vi "SV TDMS Write Octave (1 Ch).vi"(0 "tdms file":refnum<k34>, 5 "group name in":string="Octave", 7 "channel name in":string="Channel0", 9 "octave spectrum":T1, 11 "error in":errorcluster, 13 "octave info":T2={"standard"=enum."ANSI S1.11", "bandwidth"=enum."1 octave", "low band"=0, "high band"=0, "weighting filter"=0, "dB reference"=0.0, "dB On"=FALSE, "unit label"="", "channel name"="", "description"="", "engineering units"=1, "custom label"="", "spectrum type"=enum."magnitude", "spectral density"=FALSE, "filters settled"=FALSE} {"engineering units" items=["custom..."=0, "V"=1, "A"=21, "C"=30, "pC"=31, "s"=32, "-"=29, "Pa"=2, "N"=20, "g"=3, "m/s^2"=4, "m/s"=5, "m"=6, "mm/s"=12, "mm"=13, "micron/s"=14, "micron"=15, "in/s^2"=7, "in/s"=8, "in"=9, "mil/s"=10, "mil"=11, "rad/s^2"=16, "rad/s"=17, "rad"=18, "deg/s^2"=26, "deg/s"=27, "deg"=28, "RPM"=22, "cycle/s^2"=23, "Hz"=24, "cycle"=25, "strain"=19]; "dB reference" format="%.2e"; "weighting filter" items=["Linear", "A-weighting", "B-weighting", "C-weighting", "ITU-R 468-4", "Dolby", "CCITT", "C-message", "Wb", "Wc", "Wd", "We", "Wf", "Wh", "Wj", "Wk", "Wm", "AES17 20 kHz lowpass", "AES17 40 kHz lowpass", "AES17 20 kHz highpass", "AES17 40 kHz highpass"]}) -> (4 "tdms file out":refnum<k34>, 6 "group name out":string, 8 "channel name out":string, 15 "error out":errorcluster)   [LabVIEW 2017]
doc: "Writes data to the specified .tdms file in a format specific to the polymorphic instance. Wire data to the <B>scaled signal [EU]</B> input to determine the polymorphic instance to use or manually select the instance."
uses:
  <vilib>/addons/_NISVFA/_Shared subVIs/Controls/svc_Octave Info.ctl
  <vilib>/addons/_NISVFA/_Shared subVIs/Controls/svc_Octave Standard.ctl
  <vilib>/addons/_NISVFA/_Shared subVIs/Controls/svc_Weighting Filter Text Ring.ctl
  <vilib>/addons/_NISVFA/_Shared subVIs/Controls/svc_Engineering Units Text Ring.ctl
  <vilib>/addons/_NISVFA/_Shared subVIs/Controls/LV Datatypes.ctl
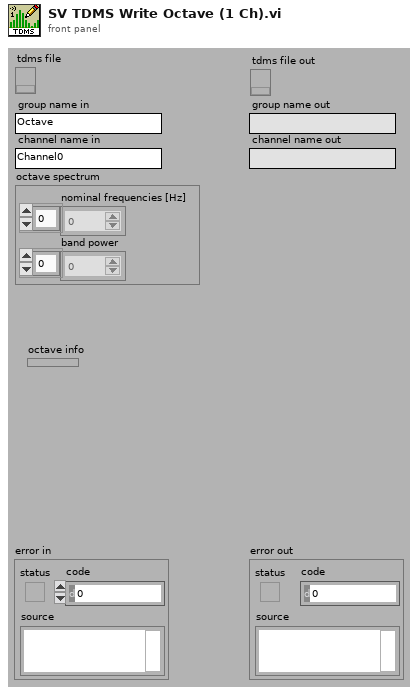
[diagram p1: front panel]
types:
  T1 = cluster{"nominal frequencies [Hz]":dbl[], "band power":dbl[]}
  T2 = typedef "svc_Octave Info.ctl" = cluster{"standard":T3, "bandwidth":enum16{"1 octave", "1/3 octave", "1/6 octave", "1/12 octave", "1/24 octave"}, "low band":i32, "high band":i32, "weighting filter":T4, "dB reference":dbl, "dB On":bool, "unit label":string, "channel name":string, "description":string, "engineering units":T5, "custom label":string, "spectrum type":enum16{"power", "magnitude"}, "spectral density":bool, "filters settled":bool}
  T3 = typedef "svc_Octave Standard.ctl" = enum16{"ANSI S1.11", "IEC 61260"}
  T4 = typedef "svc_Weighting Filter Text Ring.ctl" = u16
  T5 = typedef "svc_Engineering Units Text Ring.ctl" = u16
  T6 = typedef "LV Datatypes.ctl" = i32
  T7 = typedef "NI Function Type.ctl" = u16
  T8 = typedef "NI Function SubType.ctl" = u16
  T9 = typedef "svc_X-Axis Units.ctl" = u16
  T10 = cluster{"function type":T7, "function subtype":T8, "X-domain":T9}
  T11 = cluster{"X-axis label":string, "X-unit string":string, "Y-axis label":string, "Y-unit string":string}
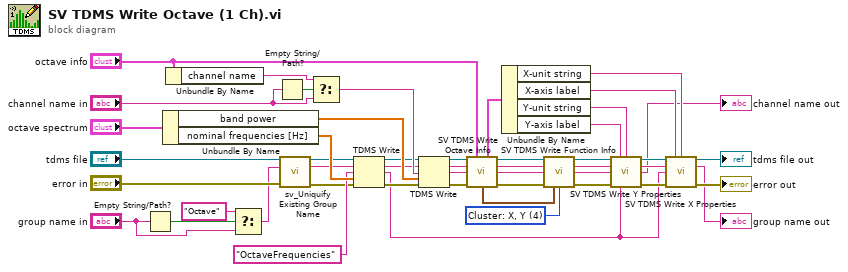
[diagram p0: block diagram]
diagram:
  w27 = T6 4 items=["String"=-2, "Boolean"=-1, "Scalar: y"=0, "Array: Y"=1, "Waveform: t0, dt, Y, variant"=2, "Cluster: x0, dx, Y"=3, "Cluster: X, Y"=4, "Waterfall"=5, "Colormap"=6] ("LabVIEW datatype")
  n1 = Empty String/Path?(string/path="group name in") -> (empty?=w4:bool)
  n2 = Unbundle By Name("octave spectrum") -> ("band power"=w43:dbl[], "nominal frequencies [Hz]"=w48:dbl[])
  n3 = Unbundle By Name("octave info") -> ("channel name"=w37:string)
  n4 = Select(t="Octave", s=w4, f="group name in") -> (s? t:f=w1:string)
  n5 = Empty String/Path?(string/path="channel name in") -> (empty?=w40:bool)
  n6 = call <vilib>:"sv_Uniquify Existing Group Name.vi"("tdms file ref"="tdms file", "group name"=w1, "error in"="error in") -> ("tdms file out"=w35:refnum<k34>, "unique group"=w34:string, "error out"=w32:errorcluster)  [unwired: 10 in]
  n7 = Select(t=w37, s=w40, f="channel name in") -> (s? t:f=w39:string)
  n8 = TDMS Write(0:w35, 5:w34, 7:"OctaveFrequencies" ("group name"), 9:w48, 11:w32) -> (4:w30:refnum<k34>, 6:w29:string, 8:w6:string, 15:w28:errorcluster)  [unwired: 1 in]
  n9 = TDMS Write(0:w30, 5:w29, 7:w39, 9:w43, 11:w28) -> (4:w46:refnum<k34>, 6:w45:string, 8:w47:string, 15:w44:errorcluster)  [unwired: 1 in]
  n10 = call <vilib>:"SV TDMS Write Octave Info.vi"("tdms file"=w46, "octave info"="octave info", "group name in"=w45, "channel name in"=w47, "error in"=w44) -> ("tdms file out"=w26:refnum<k34>, "group name out"=w25:string, "channel name out"=w24:string, "function info"=w23:T10, "unit info"=w22:T11, "error out"=w20:errorcluster)  [unwired: 5 in]
  n11 = Unbundle By Name(w22) -> ("X-unit string"=w16:string, "X-axis label"=w15:string, "Y-unit string"=w14:string, "Y-axis label"=w13:string)
  n12 = call <vilib>:"SV TDMS Write Function Info.vi"("tdms file in"=w26, "function info"=w23, "LabVIEW datatype"=w27, "group name"=w25, "channel name"=w24, "error in (no error)"=w20) -> ("tdms file out"=w17:refnum<k34>, "group name out"=w18:string, "channel name out"=w19:string, "error out"=w21:errorcluster)  [unwired: 6 in]
  n13 = call <vilib>:"SV TDMS Write Y Properties.vi"("tdms file"=w17, "y-axis label"=w13, "y-unit string"=w14, "group name"=w18, "channel name"=w19, "error in (no error)"=w21, "xchannel name"=w6) -> ("tdms file out"=w12:refnum<k34>, "group name"=w11:string, "channel name"=→"channel name out":string, "error out"=w10:errorcluster)  [unwired: 5 in]
  n14 = call <vilib>:"SV TDMS Write X Properties.vi"("tdms file in"=w12, "X-axis label"=w15, "X-unit string"=w16, "group name"=w11, "channel name"=w6, "error in"=w10) -> ("tdms file out"=→"tdms file out":refnum<k34>, "group name"=→"group name out":string, "error out"=→"error out":errorcluster)  [unwired: 6 in, 1 out]
